vi "get_number_of_retrace_pixels.vi"(8 "error in (no error)":errorcluster, 11 "DL090201FrameScanTrajectory in":refnum<class "TrajectoryDL090201FrameScan.lvclass">) -> (0 "error out":errorcluster, 2 "number of retrace pixels":i32, 3 "DL090201FrameScanTrajectory out":refnum<class "TrajectoryDL090201FrameScan.lvclass">)   [LabVIEW 2010, in "TrajectoryDL090201FrameScan.lvclass"]
uses:
  TrajectoryDL090201FrameScan.lvclass
  TrajectoryDL090201FrameScan.lvclass/TrajectoryDL090201FrameScan.ctl
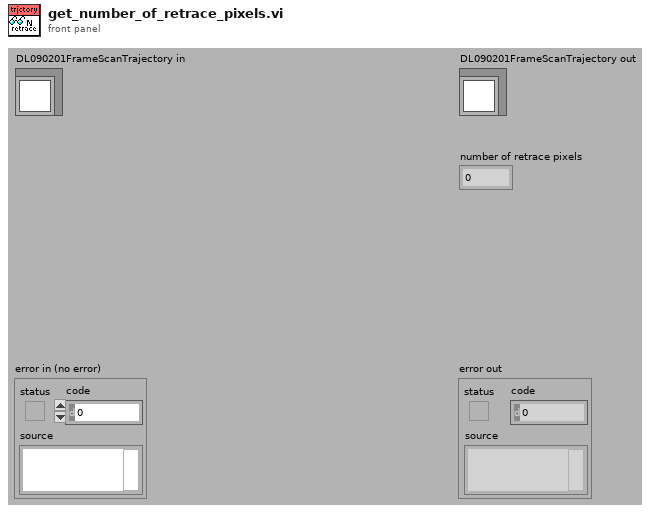
[diagram p1: front panel]
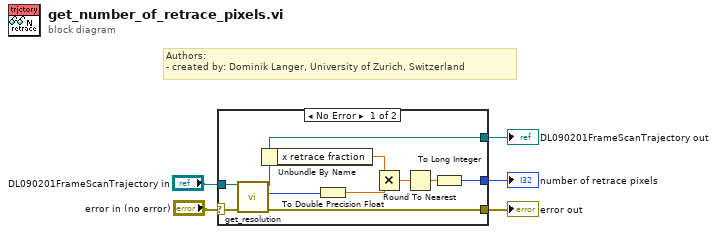
[diagram p0: block diagram]
diagram:
  # "Authors: \n- created by: Dominik Langer, University of Zurich, Switzerland"
  n1 = case shown="No Error" "error in (no error)" {
    selector: "error in (no error)" -> [w10 w17]
    tunnel: [w9 w17] -> w4
    tunnel: [w6 w16] -> w2
    tunnel: "DL090201FrameScanTrajectory in" -> [w8 w16]
    tunnel: [w11 _] -> w1
    frame No Error {
      n2 = call-dynamic "get_resolution.vi"("error in (no error)"=w10, "TrajectoryDL090201FrameScan in"=w8) -> ("error out"=w9:errorcluster, "x"=w7:i32, "TrajectoryDL090201FrameScan out"=w6:refnum<class "TrajectoryDL090201FrameScan.lvclass">)  [unwired: 7 out]
      n3 = Unbundle By Name(w6) -> ("x retrace fraction"=w14:dbl)
      n4 = To Double Precision Float(number=w7) -> (double precision float=w15:dbl)
      n5 = Multiply(x=w14, y=w15) -> (x*y=w13:dbl)
      n6 = Round To Nearest(number=w13) -> (nearest integer value=w12:dbl)
      n7 = To Long Integer(number=w12) -> (32bit integer=w11:i32)
    }
    frame Error {
    }
  }
  "error out" <- w4
  "DL090201FrameScanTrajectory out" <- w2
  "number of retrace pixels" <- w1
